vi "scrap.vi"() -> ()   [LabVIEW 2015]
uses:
  <vilib>/ptbypt/NI_PtbyPt.lvlib
panel:
  in  "file path (use dialog)":path
  in  "Waveform Controls":T1
  out "Acceleration":cluster{"all rows":dbl[], "all rows":dbl[]}(graph)
  in  "Peak Detector":T2 {"threshold valley" format="%0.2f"; "threshold peak" format="%0.2f"}
  out "Waveform Graph":dynamicdata(graph)
  out "Countrate":cluster{"Array":dbl[], dbl[]}(graph)
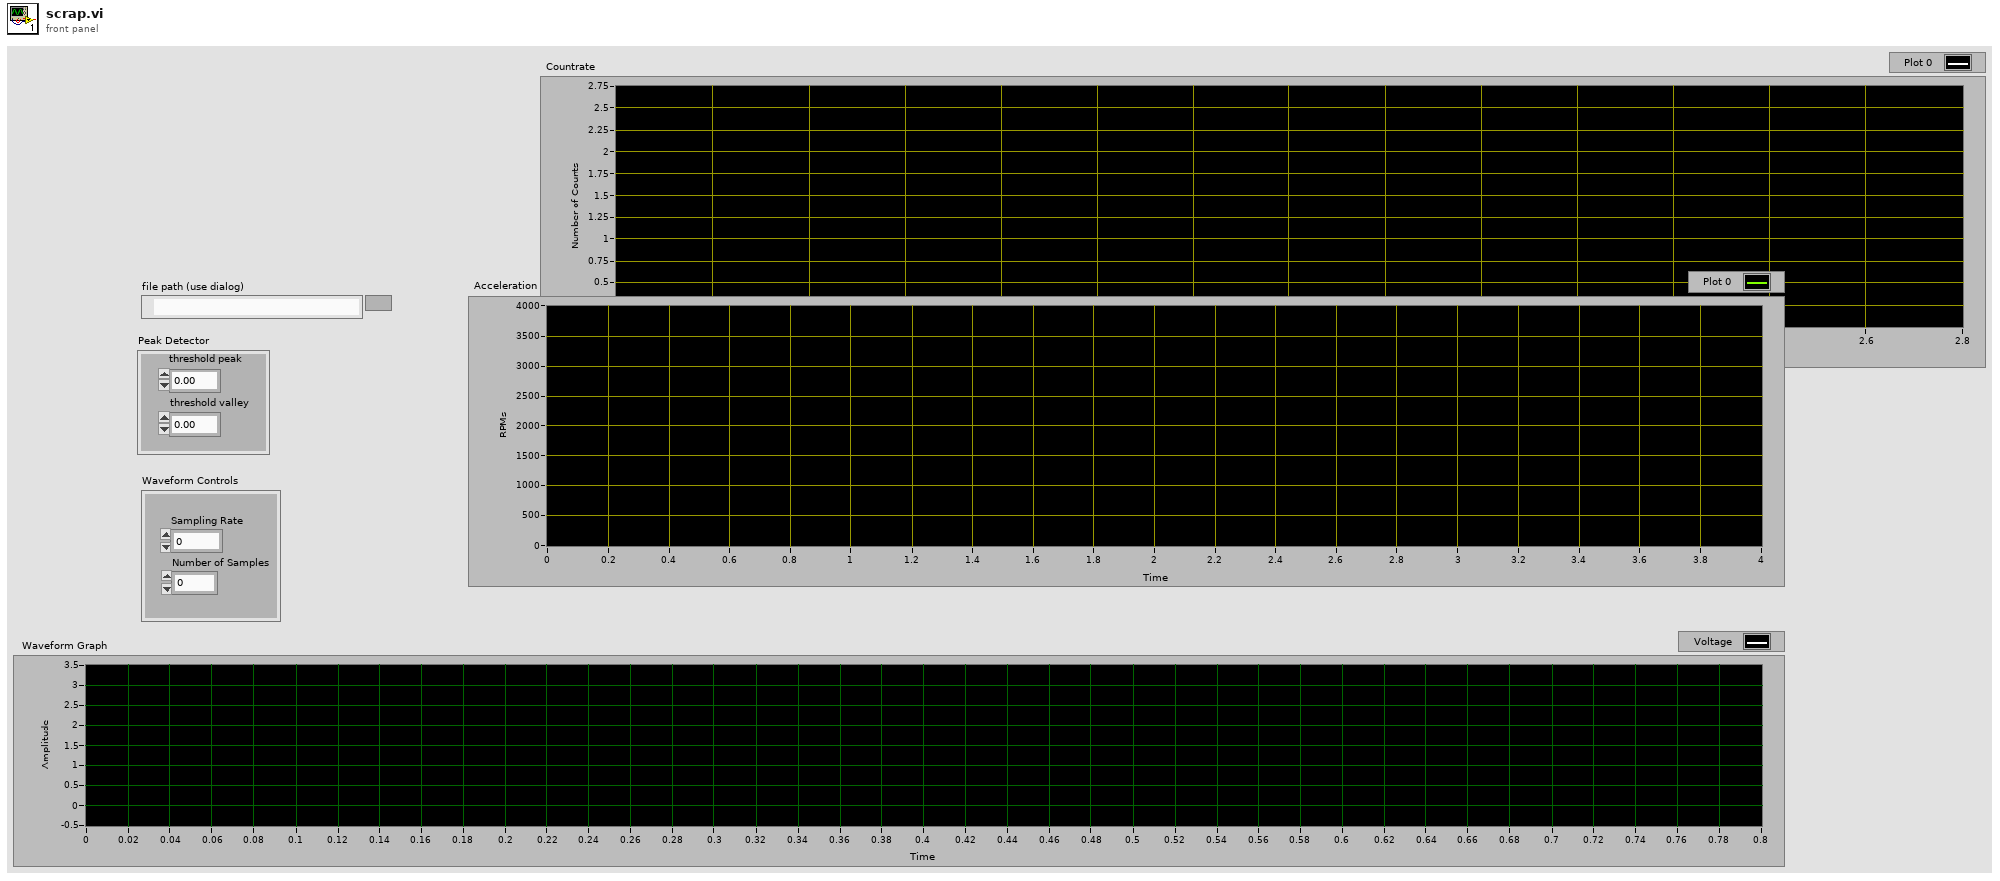
[diagram p1: front panel]
types:
  T1 = cluster{"Sampling Rate":dbl, "Number of Samples":dbl}
  T2 = cluster{"threshold peak":dbl, "threshold valley":dbl}
  T3 = enum16{"open", "replace", "create", "open or create", "replace or create", "replace or create with confirmation"}
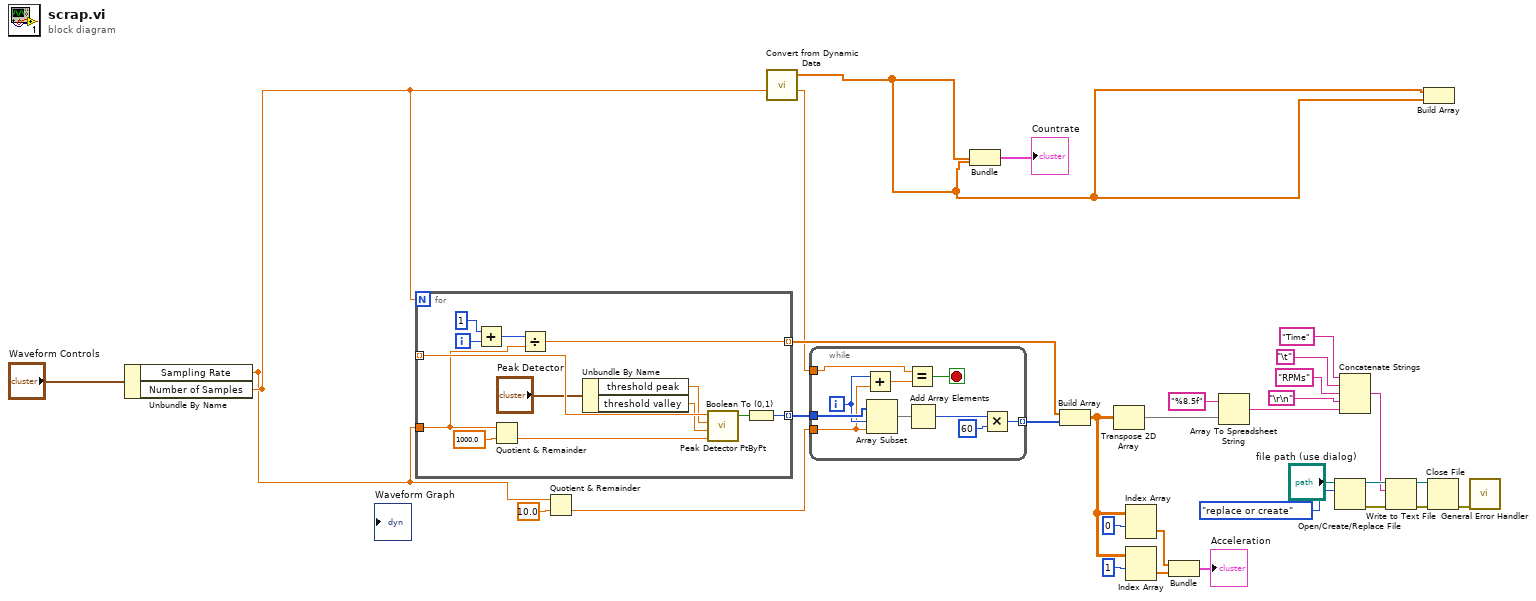
[diagram p0: block diagram]
diagram:
  n1 = Unbundle By Name("Waveform Controls") -> ("Sampling Rate"=w2:dbl, "Number of Samples"=w3:dbl)
  n2 = for {
    N: w3 -> [_]
    tunnel: w2 -> [w35]
    tunnel: [w42] -> w16 mode=indexing
    tunnel: _ -> [w41] mode=indexing
    tunnel: [w39] -> w14 mode=indexing
    i -> [w45]
    n3 = Add(x=1, y=w45) -> (x+y=w43:i32)
    n4 = Quotient & Remainder(x=w35, y=1000.0) -> (floor(x/y)=w33:dbl)  [unwired: 1 out]
    n5 = Divide(x=w43, y=w35) -> (x/y=w42:dbl)
    n6 = Unbundle By Name("Peak Detector") -> ("threshold peak"=w37:dbl, "threshold valley"=w36:dbl)
    n7 = call <vilib>:"Peak Detector PtByPt.vi"("x"=w41, "threshold peak"=w37, "threshold valley"=w36, "width"=w33) -> ("peak"=w40:bool)  [unwired: 1 in, 2 out]
    n8 = Boolean To (0,1)(Boolean=w40) -> (0, 1=w39:i16)
  }
  n9 = Quotient & Remainder(x=w2, y=10.0) -> (floor(x/y)=w11:dbl)  [unwired: 1 out]
  n10 = call "Convert from Dynamic Data"() -> ("Array"=w31:dbl[])  [unwired: 4 in]
  n11 = while {
    tunnel: w14 -> [w55]
    tunnel: [w51] -> w13 mode=indexing
    tunnel: w3 -> [w53]
    tunnel: w11 -> [w47]
    i -> [w48]
    stop <- w52 stop-if-true
    n12 = Add(x=w48, y=w47) -> (x+y=w46:dbl)
    n13 = Array Subset(array=w55, index=w48, length=w47) -> (w54:i16[])
    n14 = Equal?(x=w53, y=w46) -> (x = y?=w52:bool)
    n15 = Add Array Elements(numeric array=w54) -> (sum=w50:i16)
    n16 = Multiply(x=w50, y=60) -> (x*y=w51:i32)
  }
  n17 = Bundle("Array"=w31, "Array"=w31) -> (→"Countrate":cluster{"Array":dbl[], "Array":dbl[]})  [unwired: 1 in]
  n18 = Build Array(w16, w13) -> (w5:dbl[][])
  n19 = Transpose 2D Array(2D array=w5) -> (transposed array=w15:dbl[][])
  n20 = Index Array(array=w5, index (row)=0 ("index")) -> (element=w8:dbl[])  [unwired: 1 in]
  n21 = Index Array(array=w5, index (row)=1 ("index")) -> (element=w7:dbl[])  [unwired: 1 in]
  n22 = Bundle(w8, w7) -> (→"Acceleration":cluster{dbl[], dbl[]})  [unwired: 1 in]
  n23 = Array To Spreadsheet String(array=w15, 3:"%8.5f" ("format string")) -> (spreadsheet string=w19:string)  [unwired: 1 in]
  n24 = Open/Create/Replace File(file path (use dialog)="file path (use dialog)", operation (0:open)=T3."replace or create") -> (refnum out=w27:refnum<file>, error out=w28:errorcluster)  [unwired: 4 in, 1 out]
  n25 = Concatenate Strings("Time" ("string"), "\t", "RPMs" ("string"), "\r\n", w19) -> (w18:string)
  n26 = Write to Text File(file (use dialog)=w27, text=w18, error in=w28) -> (refnum out=w26:refnum<file>, error out=w29:errorcluster)  [unwired: 1 in, 1 out]
  n27 = Build Array(w31, w31) -> ()  [unwired: 1 out]
  n28 = Close File(refnum=w26, error in=w29) -> (error out=w30:errorcluster)  [unwired: 1 out]
  n29 = call <vilib>:"General Error Handler.vi"("error in (no error)"=w30) -> ()  [unwired: 10 in, 5 out]
